vi "Get Module Mode.vi"(8 "error in (no error)":errorcluster, 11 "module in":refnum<class "Module.lvclass">) -> (0 "error out":errorcluster, 1 "module mode":string, 2 "module name":string, 3 "module out":refnum<class "Module.lvclass">)   [LabVIEW 2019, in "Scan Engine Example Support.lvlib"]
uses:
  Scan Engine Example Support.lvlib
  <vilib>/addons/VeriStand Custom Device Scripting APIs/Scan Engine/Modules/Module/Module.lvclass
  <vilib>/addons/VeriStand Custom Device Scripting APIs/Scan Engine/Modules/Mode Classes/Mode/Mode.lvclass
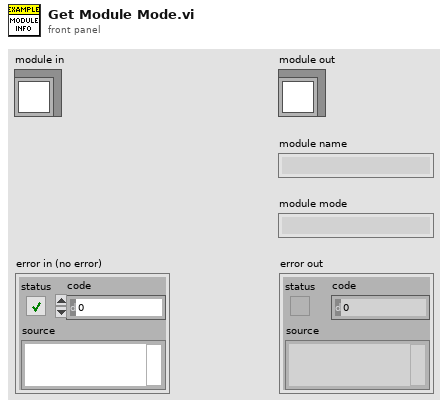
[diagram p1: front panel]
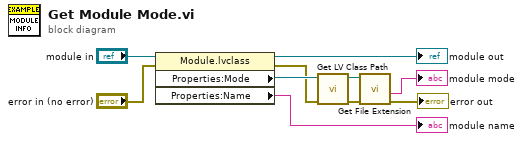
[diagram p0: block diagram]
diagram:
  n1 = property class="Module.lvclass"(reference="module in", error in="error in (no error)") -> (reference out=→"module out":refnum<class "Module.lvclass">, error out=w6:errorcluster, "Properties:Mode"=w9:refnum<class "Mode.lvclass">, "Properties:Name"=→"module name":string)
  n2 = call <vilib>:"Get LV Class Path.vi"("error in (no error)"=w6, "object"=w9) -> ("error out"=w5:errorcluster, "class path"=w10:path)  [unwired: 8 in]
  n3 = call <vilib>:"Get File Extension.vi"("error in (no error)"=w5, "file"=w10) -> ("error out"=→"error out":errorcluster, "filename without extension"=→"module mode":string)  [unwired: 5 in, 3 out]
